vi "EnFlo_Seeder_Control.vi"(0 "Current Time (s)":dbl) -> ()   [LabVIEW 2014]
panel:
  in  "Minium Seeder power setting (Pmin)":dbl=27.0
  in  "Minimum Transducer Setting (Tmin)":dbl=6.0
  in  "Fluid Flowrate Factor":dbl=1.2 min=0.2 max=4.0 step=0.1 format="%.1g"
  in  "Sugar Strength":dbl=0.23
  out "Leak Detected or Emergency Stop":bool
  in  "Performing hand clean":bool
  out "Run Transducer":bool
  out "Sugar Pump":bool
  out "Low Flow":bool
  out "High Flow":bool
  out "Time Since Last Flush (min)":dbl
  out "Running Flush time":dbl
  out "Transducer setting":dbl
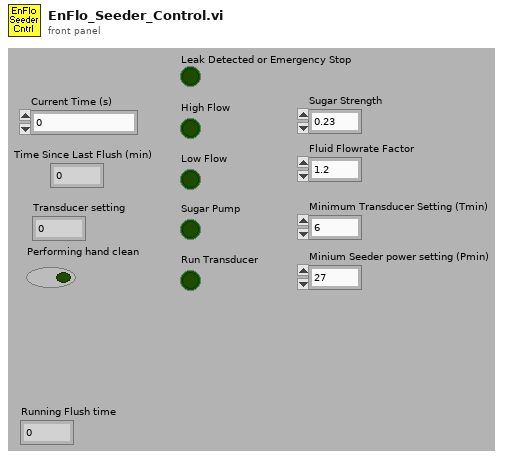
[diagram p1: front panel]
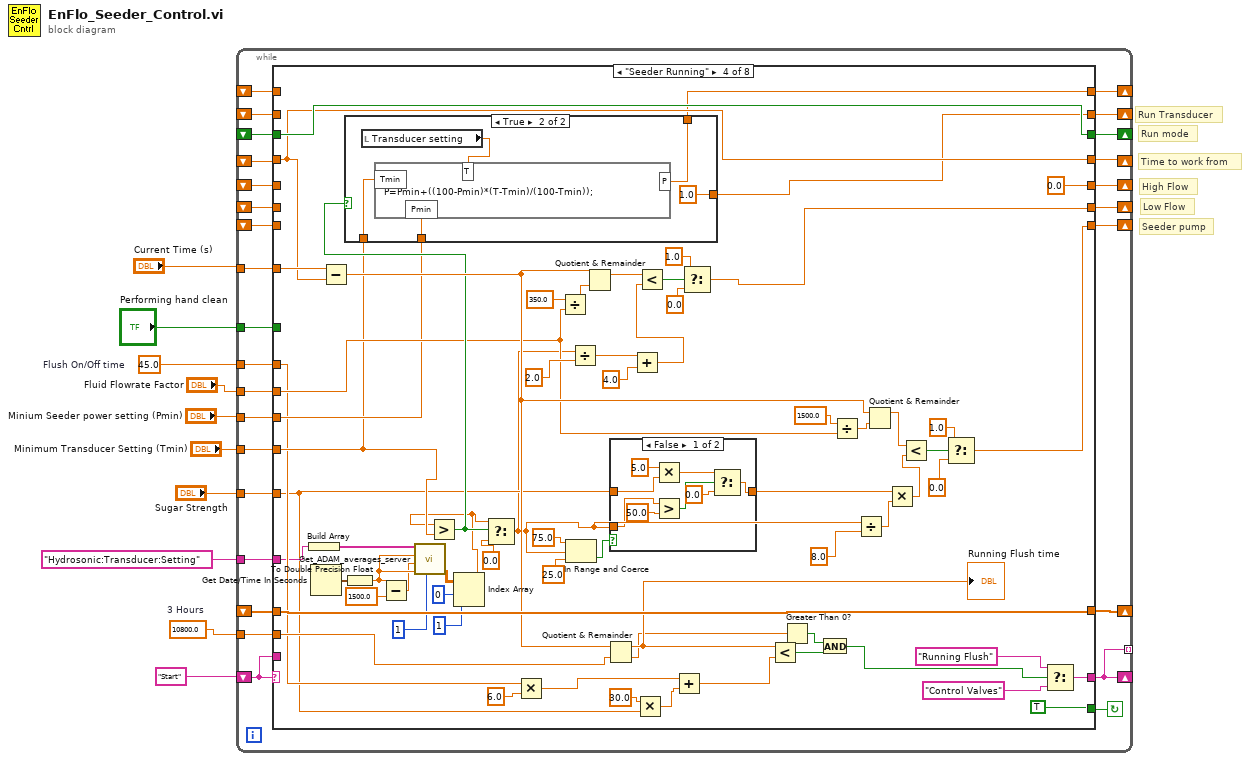
[diagram p0: block diagram]
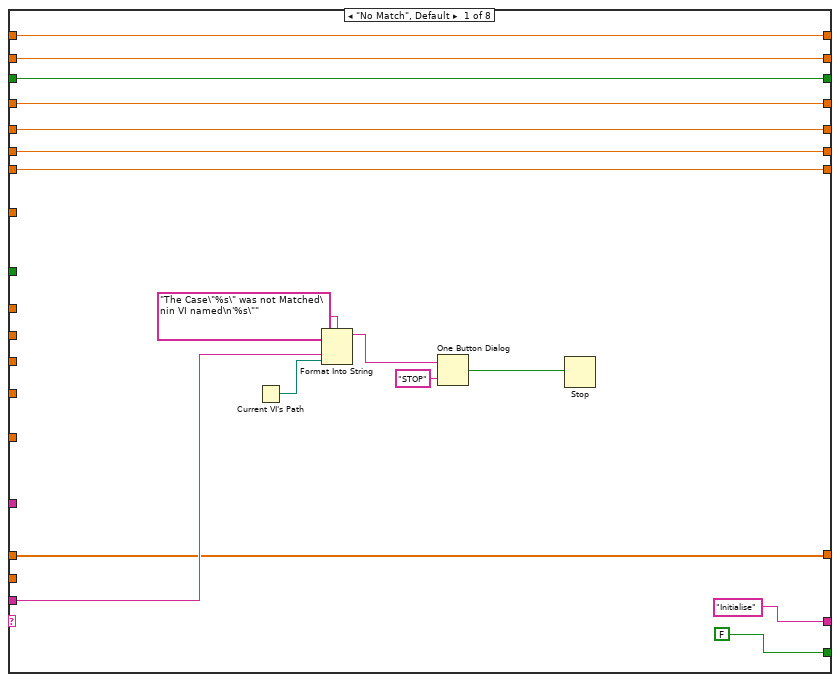
[diagram p2: hidden frame]
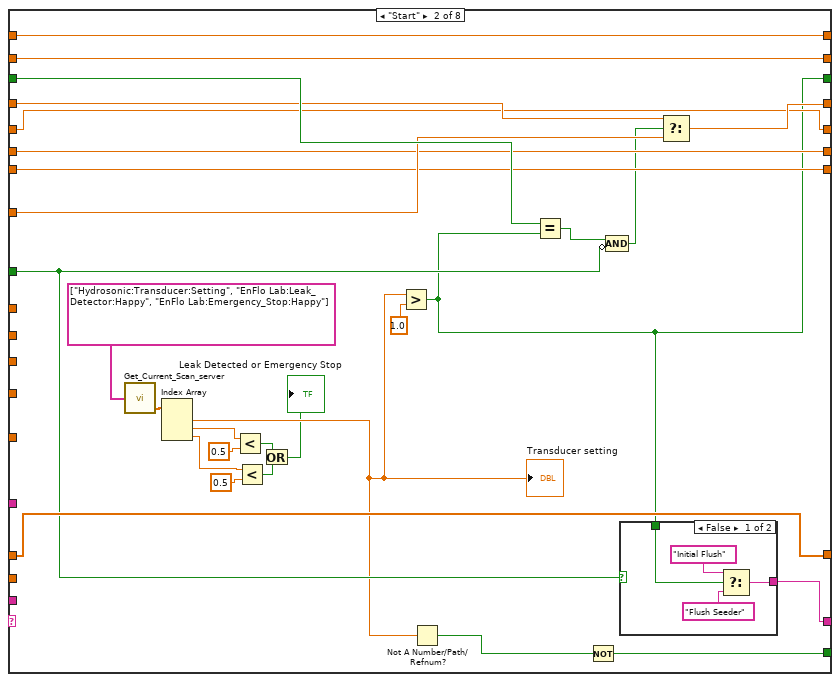
[diagram p3: hidden frame]
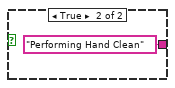
[diagram p4: hidden frame]
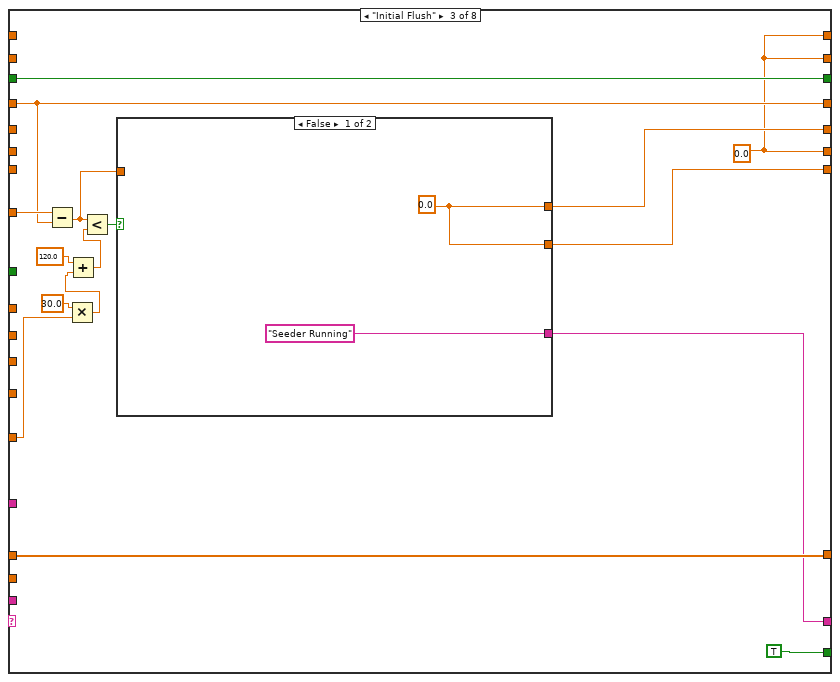
[diagram p5: hidden frame]
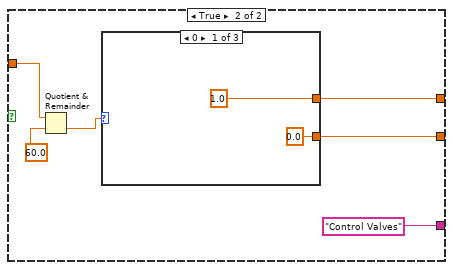
[diagram p6: hidden frame]
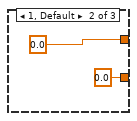
[diagram p7: hidden frame]
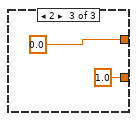
[diagram p8: hidden frame]
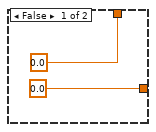
[diagram p10: hidden frame]
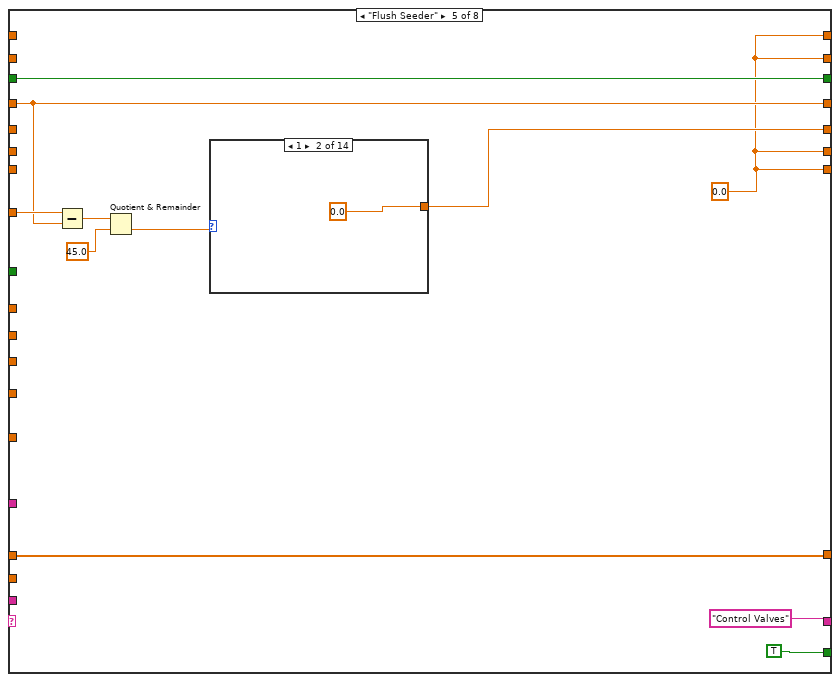
[diagram p11: hidden frame]
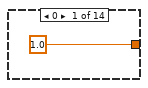
[diagram p12: hidden frame]
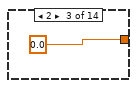
[diagram p13: hidden frame]
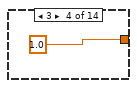
[diagram p14: hidden frame]
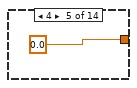
[diagram p15: hidden frame]
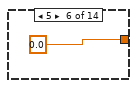
[diagram p16: hidden frame]
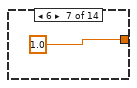
[diagram p17: hidden frame]
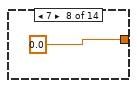
[diagram p18: hidden frame]
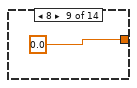
[diagram p19: hidden frame]
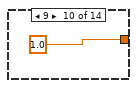
[diagram p20: hidden frame]
diagram:
  w2 = 45.0  # Flush On/Off time
  w8 = 10800.0  # 3 Hours
  # "Run Transducer"
  # "Seeder pump"
  # "Low Flow"
  # "High Flow"
  # "Run mode"
  # "Time to work from"
  n1 = while {
    shift-left: "Start" -> [w37]
    shift-right: [w21] -> _
    shift-right: [w36] -> _
    shift-left: _ -> [w33]
    shift-right: [w35] -> _
    shift-left: _ -> [w34]
    tunnel: "Current Time (s)" -> [w32]
    shift-right: [w30] -> _
    shift-left: _ -> [w31]
    shift-right: [w29] -> _
    shift-left: _ -> [w28]
    shift-right: [w26] -> _
    shift-left: _ -> [w27]
    shift-right: [w24] -> _
    shift-left: _ -> [w25]
    shift-right: [w23] -> _
    shift-left: _ -> [w22]
    tunnel: [w21] -> _ mode=indexing
    tunnel: w8 -> [w20]
    tunnel: "Performing hand clean" -> [w19]
    tunnel: "Sugar Strength" -> [w18]
    shift-right: [w17] -> _
    shift-left: _ -> [w16]
    tunnel: "Fluid Flowrate Factor" -> [w15]
    tunnel: "Minimum Transducer Setting (Tmin)" -> [w14]
    tunnel: "Minium Seeder power setting (Pmin)" -> [w13]
    tunnel: w2 -> [w12]
    tunnel: "Hydrosonic:Transducer:Setting" -> [w11]
    stop <- w38 continue-if-true
    n2 = case shown="\"Seeder Running\"" w37 {
      tunnel: [FALSE w80 TRUE TRUE TRUE TRUE TRUE FALSE] -> w38
      tunnel: ["Initialise" w75 w94 w163 "Control Valves" "Control Valves" "Control Valves" "End"] -> w21
      tunnel: w37 -> [w49 _ _ _ _ _ _ _]
      tunnel: [w44 w78 w97 w182 w207 w228 w242 w295] -> w36
      tunnel: [w46 w60 w102 w184 w209 w229 w243 w304] -> w35
      tunnel: w34 -> [w46 w79 w102 w184 w209 w229 w243 w304]
      tunnel: w33 -> [w44 w77 w97 w182 w207 w228 w242 w295]
      tunnel: w32 -> [_ w76 w98 w183 w208 _ _ w296]
      tunnel: w31 -> [w45 w74 _ _ _ _ _ w292]
      tunnel: [w45 w74 w101 0.0 w203 w226 w241 w292] -> w30
      tunnel: w28 -> [w43 w72 _ _ _ _ _ w290]
      tunnel: [w43 w72 w88 w172 w201 w226 w237 w290] -> w29
      tunnel: w27 -> [w42 w71 _ _ _ _ _ w288]
      tunnel: [w42 w71 w99 w166 w201 w226 w238 w288] -> w26
      tunnel: w25 -> [w41 w73 w100 w181 w202 w227 w240 w284]
      tunnel: [w41 w73 w100 w181 w202 w227 w240 w277] -> w24
      tunnel: w22 -> [w40 w70 _ _ _ _ _ w286]
      tunnel: [w40 w70 w88 w147 w201 w226 w237 w286] -> w23
      tunnel: w20 -> [_ _ _ w155 _ _ _ w280]
      tunnel: w19 -> [_ w67 _ _ _ _ _ _]
      tunnel: w18 -> [_ _ w91 w122 _ _ _ _]
      tunnel: [w39 w63 w88 w146 w201 w226 w237 w272] -> w17
      tunnel: w16 -> [w39 w63 _ _ _ _ _ w272]
      tunnel: w15 -> [_ _ _ w141 _ _ _ _]
      tunnel: w14 -> [_ _ _ w138 _ _ _ _]
      tunnel: w13 -> [_ _ _ w139 _ _ _ _]
      tunnel: w12 -> [_ _ _ w137 _ _ w236 _]
      tunnel: w11 -> [_ _ _ w134 _ _ _ _]
      frame "No Match", Default {
        n3 = Current VI's Path() -> (path=w48:path)
        n4 = Format Into String(format string="The Case\"%s\" was not Matched\nin VI named\n'%s\"" ("Format String"), w49, w48) -> (resulting string=w52:string)  [unwired: 2 in, 1 out]
        n5 = One Button Dialog(message=w52, button name ("OK")="STOP") -> (true=w50:bool)
        n6 = Stop(stop? (T)=w50) -> ()
      }
      frame "Start" {
        n7 = call "Get_Current_Scan_server.vi"("Desired Channels"=string[] ["Hydrosonic:Transducer:Setting", "EnFlo Lab:Leak_Detector:Happy", "EnFlo Lab:Emergency_Stop:Happy"] ("appended array")) -> ("Numerical Values"=w82:dbl[])  [unwired: 2 out]
        n8 = Index Array(array=w82) -> (element #1=w62:dbl, element #2=w65:dbl, element #3=w58:dbl)  [unwired: 3 in]
        "Transducer setting" <- w62
        n9 = Less?(x=w65, y=0.5) -> (x < y?=w56:bool)
        n10 = Less?(x=w58, y=0.5) -> (x < y?=w57:bool)
        n11 = Or(x=w56, y=w57) -> (x .or. y?=→"Leak Detected or Emergency Stop":bool)
        n12 = Greater?(x=w62, y=1.0) -> (0:w60:bool)
        n13 = Not A Number/Path/Refnum?(number/path/refnum=w62) -> (NaN/Path/Refnum?=w81:bool)
        n14 = Equal?(x=w79, y=w60) -> (x = y?=w69:bool)
        n15 = Not(x=w81) -> (.not. x?=w80:bool)
        n16 = Compound Arithmetic op=AND(w69, invert w67) -> (w68:bool)
        n17 = case shown="False" w67 {
          tunnel: w60 -> [w86 _]
          tunnel: [w85 "Performing Hand Clean"] -> w75
          frame False {
            n18 = Select(t="Initial Flush", s=w86, f="Flush Seeder") -> (s? t:f=w85:string)
          }
          frame True {
          }
        }
        n19 = Select(t=w77, s=w68, f=w76) -> (s? t:f=w78:dbl)
      }
      frame "Initial Flush" {
        w88 = 0.0
        n20 = Subtract(x=w98, y=w97) -> (x-y=w95:dbl)
        n21 = Multiply(x=30.0 ("y"), y=w91) -> (x*y=w90:dbl)
        n22 = Add(x=120.0 ("y"), y=w90) -> (x+y=w89:dbl)
        n23 = Less?(x=w95, y=w89) -> (x < y?=w96:bool)
        n24 = case shown="False" w96 {
          tunnel: [w105 w111] -> w101
          tunnel: [w105 w110] -> w99
          tunnel: w95 -> [_ w108]
          tunnel: ["Seeder Running" "Control Valves"] -> w94
          frame False {
            w105 = 0.0
          }
          frame True {
            n25 = Quotient & Remainder(x=w108, y=60.0) -> (floor(x/y)=w107:dbl)  [unwired: 1 out]
            n26 = case shown="0" w107 {
              tunnel: [1.0 0.0 0.0] -> w111
              tunnel: [0.0 0.0 1.0] -> w110
              frame 0 {
              }
              frame 1, Default {
              }
              frame 2 {
              }
            }
          }
        }
      }
      frame "Seeder Running" {
        n27 = Build Array(w134) -> (w133:string[])
        n28 = Get Date/Time In Seconds() -> (seconds since 1Jan1904=w132:timestamp)
        n29 = Subtract(x=w183, y=w182) -> (x-y=w161:dbl)
        n30 = To Double Precision Float(number=w132) -> (double precision float=w131:dbl)
        n31 = Subtract(x=w131, y=1500.0) -> (x-y=w118:dbl)
        n32 = call "Get_ADAM_averages_server.vi"("No of averages"=1, "End time"=w131, "Start time"=w118, "Clients time"=w131, "ADAM Ch Names"=w133) -> ("DBL values"=w129:dbl[][])  [unwired: 1 in, 4 out]
        n33 = Index Array(array=w129, index (row)=0, index (col)=1 ("disabled index (col)")) -> (element=w126:dbl)
        n34 = Greater?(x=w126, y=w138) -> (0:w148:bool)
        n35 = case shown="True" w148 {
          tunnel: [0.0 1.0] -> w147
          tunnel: [0.0 w197] -> w146
          tunnel: w139 -> [_ w199]
          tunnel: w138 -> [_ w198]
          frame False {
          }
          frame True {
            n36 = local read "Transducer setting"() -> (w196:dbl)
            n37 = formula code="P=Pmin+((100-Pmin)*(T-Tmin)/(100-Tmin));"("Tmin"=w198, "T"=w196, "Pmin"=w199) -> ("P"=w197:dbl)
          }
        }
        n38 = Select(t=w126, s=w148, f=0.0) -> (s? t:f=w120:dbl)
        n39 = Multiply(x=w137, y=6.0) -> (x*y=w135:dbl)
        n40 = Divide(x=350.0 ("y"), y=w141) -> (x/y=w143:dbl)
        n41 = In Range and Coerce(upper limit=75.0, x=w120, lower limit=25.0) -> (In Range?=w123:bool)  [unwired: 1 out]
        n42 = Divide(x=w120, y=2.0) -> (x/y=w145:dbl)
        n43 = Quotient & Remainder(x=w161, y=w143) -> (x-y*floor(x/y)=w180:dbl)  [unwired: 1 out]
        n44 = Quotient & Remainder(x=w161, y=w155) -> (x-y*floor(x/y)=w162:dbl, floor(x/y)=w159:dbl)
        "Running Flush time" <- w162
        n45 = case shown="False" w123 {
          tunnel: w122 -> [w186 w193]
          tunnel: [w190 w193] -> w121
          tunnel: w120 -> [w192 _]
          frame False {
            n46 = Multiply(x=5.0, y=w186) -> (x*y=w187:dbl)
            n47 = Greater?(x=w192, y=50.0) -> (0:w189:bool)
            n48 = Select(t=w187, s=w189, f=0.0) -> (s? t:f=w190:dbl)
          }
          frame True {
          }
        }
        n49 = Add(x=w145, y=4.0) -> (x+y=w175:dbl)
        n50 = Multiply(x=30.0 ("y"), y=w122) -> (x*y=w151:dbl)
        n51 = Less?(x=w180, y=w175) -> (x < y?=w179:bool)
        n52 = Add(x=w135, y=w151) -> (x+y=w150:dbl)
        n53 = Select(t=1.0, s=w179, f=0.0) -> (s? t:f=w172:dbl)
        n54 = Less?(x=w162, y=w150) -> (x < y?=w157:bool)
        n55 = Greater Than 0?(x=w159) -> (x > 0?=w158:bool)
        n56 = And(x=w158, y=w157) -> (x .and. y?=w156:bool)
        n57 = Divide(x=1500.0 ("y"), y=w141) -> (x/y=w140:dbl)
        n58 = Divide(x=w120, y=8.0) -> (x/y=w153:dbl)
        n59 = Quotient & Remainder(x=w161, y=w140) -> (x-y*floor(x/y)=w167:dbl)  [unwired: 1 out]
        n60 = Multiply(x=w121, y=w153) -> (x*y=w154:dbl)
        n61 = Less?(x=w167, y=w154) -> (x < y?=w168:bool)
        n62 = Select(t=1.0, s=w168, f=0.0) -> (s? t:f=w166:dbl)
        n63 = Select(t="Running Flush", s=w156, f="Control Valves") -> (s? t:f=w163:string)
      }
      frame "Flush Seeder" {
        w201 = 0.0
        n64 = Subtract(x=w208, y=w207) -> (x-y=w206:dbl)
        n65 = Quotient & Remainder(x=w206, y=45.0) -> (floor(x/y)=w204:dbl)  [unwired: 1 out]
        n66 = case shown="1" w204 {
          tunnel: [1.0 0.0 0.0 1.0 0.0 0.0 1.0 0.0 0.0 1.0 0.0 0.0 1.0 0.0] -> w203
          frame 0 {
          }
          frame 1 {
          }
          frame 2 {
          }
          frame 3 {
          }
          frame 4 {
          }
          frame 5 {
          }
          frame 6 {
          }
          frame 7 {
          }
          frame 8 {
          }
          frame 9 {
          }
          frame 10 {
          }
          frame 11 {
          }
          frame 12 {
          }
          frame 13, Default {
          }
        }
      }
      frame "Performing Hand Clean" {
        w226 = 0.0
      }
      frame "Running Flush" {
        w237 = 0.0
        n67 = local read "Running Flush time"() -> (w239:dbl)
        n68 = Quotient & Remainder(x=w239, y=w236) -> (floor(x/y)=w235:dbl)  [unwired: 1 out]
        n69 = To Long Integer(number=w235) -> (32bit integer=w232:i32)
        n70 = feedback-in #1(w232) -> ()
        n71 = feedback #1() -> (w234:i32)  [unwired: 1 in]
        n72 = Not Equal?(x=w232, y=w234) -> (x != y?=w233:bool)
        n73 = case shown="0" w232 {
          tunnel: [1.0 0.0 1.0 0.0 1.0 0.0 0.0] -> w241
          tunnel: [0.0 0.0 0.0 0.0 0.0 0.0 1.0] -> w238
          tunnel: w233 -> [_ _ _ _ _ _ w258]
          frame 0 {
          }
          frame 1 {
          }
          frame 2 {
          }
          frame 3 {
          }
          frame 4 {
          }
          frame 5, Default {
          }
          frame 6 {
            n74 = local read "Transducer setting"() -> (w261:dbl)
            n75 = In Range and Coerce(upper limit=90.0, x=w261, lower limit=8.0) -> (In Range?=w259:bool)  [unwired: 1 out]
            n76 = And(x=w259, y=w258) -> (x .and. y?=w260:bool)
            n77 = case shown="True" w260 {
              tunnel: w261 -> [_ w269]
              frame False {
              }
              frame True {
                n78 = Add(x=w269, y=10.0) -> (x+y=w266:dbl)
                n79 = Build Array("Hydrosonic:Transducer:Setting") -> (w270:string[])
                n80 = Build Array(w266) -> (w267:dbl[])
                n81 = call "ASYNC_Adam_server.vi"("Values"=w267, "Channel Names"=w270) -> ()  [unwired: 1 in, 3 out]
              }
            }
          }
        }
      }
      frame "Control Valves" {
        n82 = Subtract(x=w296, y=w295) -> (x-y=w281:dbl)
        n83 = local read "Leak Detected or Emergency Stop"() -> (w278:bool)
        n84 = Quotient & Remainder(x=w281, y=w280) -> (x-y*floor(x/y)=w279:dbl)  [unwired: 1 out]
        n85 = Divide(x=w279, y=60.0) -> (x/y=→"Time Since Last Flush (min)":dbl)
        n86 = Build Array(w286, w292, w290, w288, w272) -> (w274:dbl[])
        n87 = Array Size(array=w284) -> (size(s)=w283:i32)
        n88 = Equal To 0?(x=w283) -> (x = 0?=w282:bool)
        n89 = Array Size(array=w274) -> (size(s)=w276:i32)
        n90 = Initialize Array(0.0 ("element"), w276) -> (w273:dbl[])
        n91 = Select(t=w273, s=w278, f=w274) -> (s? t:f=w277:dbl[])
        n92 = case shown="False" w282 {
          tunnel: w277 -> [w309 w314]
          tunnel: string[] ["Hydrosonic:Seeder:Enable", "EnFlo_Tunnel:Seeder:High_Flow", "EnFlo_Tunnel:Seeder:Low_Flow", "EnFlo_Tunnel:Seeder_Pump:Enable", "EnFlo_Tunnel:Seeder:Power"] ("Desired Ch Names") -> [w308 w315]
          tunnel: [w307 w315] -> w300
          tunnel: [w306 w314] -> w299
          tunnel: w284 -> [w305 _]
          frame False {
            n93 = for {
              tunnel: w305 -> [w313] mode=indexing
              tunnel: w309 -> [w312] mode=indexing
              tunnel: [w312] -> w306 mode=indexing if=w310
              tunnel: w308 -> [w311] mode=indexing
              tunnel: [w311] -> w307 mode=indexing if=w310
              n94 = Not Equal?(x=w312, y=w313) -> (x != y?=w310:bool)
            }
          }
          frame True {
          }
        }
        n95 = Array Size(array=w299) -> (size(s)=w303:i32)
        n96 = Greater Than 0?(x=w303) -> (x > 0?=w302:bool)
        n97 = case shown="True" w302 {
          tunnel: w299 -> [_ w317]
          tunnel: w300 -> [_ w316]
          frame False {
          }
          frame True {
            n98 = call "ASYNC_Adam_server.vi"("Values"=w317, "Channel Names"=w316) -> ()  [unwired: 1 in, 3 out]
          }
        }
        n99 = Greater Than 0?(x=w292) -> (x > 0?=→"High Flow":bool)
        n100 = Greater Than 0?(x=w290) -> (x > 0?=→"Low Flow":bool)
        n101 = Greater Than 0?(x=w286) -> (x > 0?=→"Run Transducer":bool)
        n102 = Greater Than 0?(x=w288) -> (x > 0?=→"Sugar Pump":bool)
      }
    }
  }
